vi "socket.vi"(8 "error in (no error)":errorcluster) -> (0 "error out":errorcluster, 3 "tcp socket fd":i32)   [LabVIEW 2015]
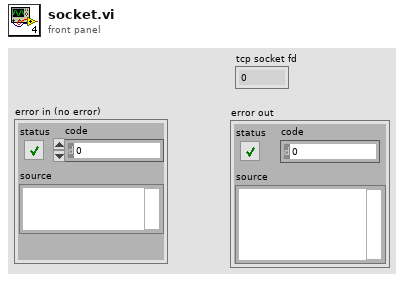
[diagram p1: front panel]
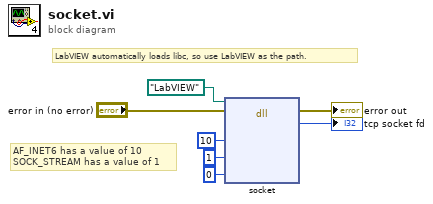
[diagram p0: block diagram]
diagram:
  # "LabVIEW automatically loads libc, so use LabVIEW as the path."
  # "AF_INET6 has a value of 10\nSOCK_STREAM has a value of 1"
  n1 = dll-call lib="LabVIEW" fn="socket"(path in=path "LabVIEW", error in="error in (no error)", "domain"=u16 10, "type"=u16 1, "protocol"=u16 0) -> (error out=→"error out":errorcluster, "tcp socket"=→"tcp socket fd":i32)  [unwired: 4 in, 1 out]
